vi "xiCam - Get1DImageData_ExternalDimension.vi"(7 "timeout":i32, 8 "error in (no error)":errorcluster, 9 "1DImageData In":u8[](array[numeric]), 11 "xiCam In":refnum<k24>) -> (0 "error out":errorcluster, 1 "1DImageData Out":u8[](array[numeric]), 3 "xiCam Out":refnum<k24>)   [LabVIEW 2015]
doc: "This function acquires image and returns a preallocated byte array containing the Image data.\n\n<b>void GetImage(byte* ImageData, int timeout)</b>\nint timeout : Time interval required to wait for the image (in milliseconds)"
uses:
  C:/GIT/Cameras3.x/Integrations/Labview/xiLib/xiLIB_32bit/xiLIB/xiCamLib/API/x86/xiApi.NET.dll
  xiLIB_32bit/xiLIB/xiCamLib/API/x86/xiApi.NET.dll
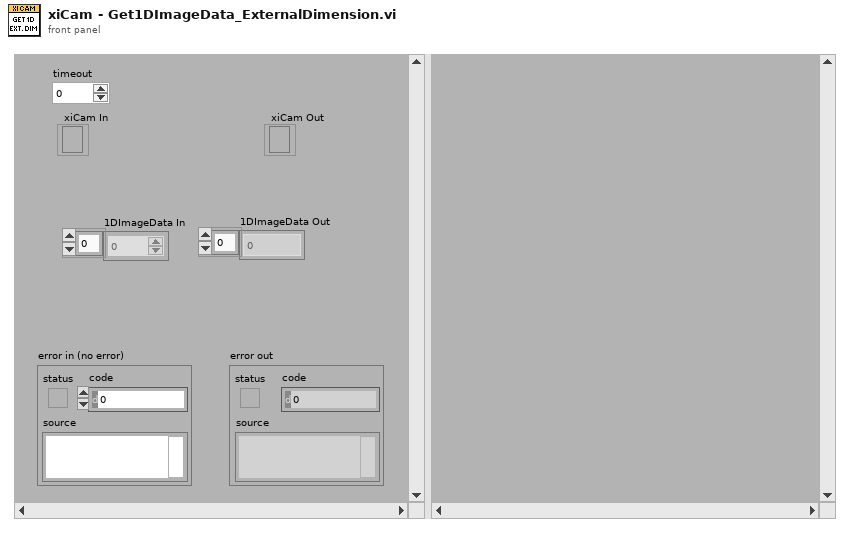
[diagram p1: front panel]
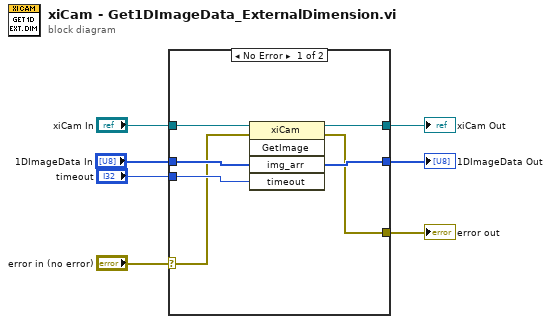
[diagram p0: block diagram]
diagram:
  n1 = case shown="No Error" "error in (no error)" {
    selector: "error in (no error)" -> [w8 w15]
    tunnel: "xiCam In" -> [w14 w16]
    tunnel: [w13 w16] -> w5
    tunnel: [w10 w15] -> w4
    tunnel: "timeout" -> [w12 _]
    tunnel: [w11 _] -> w2
    tunnel: "1DImageData In" -> [w9 _]
    frame No Error {
      n2 = invoke class="xiCam" method="GetImage"(reference=w14, error in=w8, "img_arr"=w9, "timeout"=w12) -> (reference out=w13:refnum<k24>, error out=w10:errorcluster, "img_arr"=w11:u8[])  [unwired: 1 in, 2 out]
    }
    frame Error {
    }
  }
  "error out" <- w4
  "xiCam Out" <- w5
  "1DImageData Out" <- w2
